vi "LEM_Paramters.vi"(8 "error in":errorcluster, 11 "Model Data":T2 {"Matricies"."K" format="%#_6e"; "Matricies"."Dout" format="%#_6e"; "Matricies"."Bout" format="%#_6e"; "Matricies"."Aout" format="%#_6e"; "Matricies"."Dint" format="%#_6e"; "Matricies"."Bint" format="%#_6e"; "Matricies"."Aint" format="%#_6e"; "Constants"."Z" format="%^#_6e"}) -> (0 "error out":errorcluster, 3 "Model Data Out":T2 {"Matricies"."K" format="%#_6e"; "Matricies"."Dout" format="%#_6e"; "Matricies"."Bout" format="%#_6e"; "Matricies"."Aout" format="%#_6e"; "Matricies"."Dint" format="%#_6e"; "Matricies"."Bint" format="%#_6e"; "Matricies"."Aint" format="%#_6e"; "Constants"."Z" format="%^#_6e"})   [LabVIEW 2022 SP3]
uses:
  Model Data.ctl
  PZT type.ctl
  Piezo_Discs.ctl
  LEM_Params.ctl
  Layer Properties.ctl
  Matricies.ctl
  <vilib>/Utility/error.llb/DialogType.ctl
  <vilib>/Analysis/2dsp.llb/Integral Method.ctl
  <vilib>/Analysis/8numeric.llb/1D Numeric Integration.vi
  <vilib>/Analysis/NI_AALPro.lvlib
panel:
  out "LEM Parameters":T1
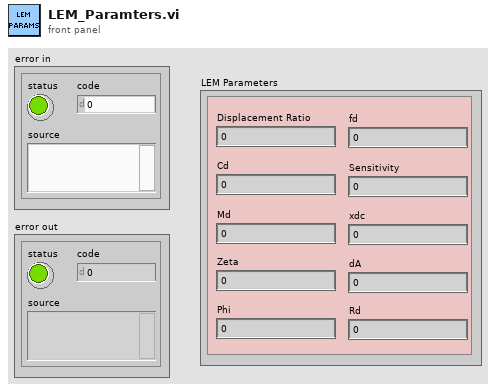
[diagram p1: front panel]
types:
  T1 = typedef "LEM_Params.ctl" = cluster{"Displacement Ratio":dbl, "Cd":dbl, "Md":dbl, "xdc":dbl, "fd":dbl, "Sensitivity":dbl, "dA":dbl, "Rd":dbl, "Zeta":dbl, "Phi":dbl}
  T2 = typedef "Model Data.ctl" = cluster{"Disc Properties":cluster{"Type":T3, "Disc Model":T4}, "Constants":cluster{"Radius":dbl[], "U(r)":dbl[], "W(r)":dbl[], "Vac":dbl, "P":dbl, "RiRo":dbl, "Area Density (r)":dbl[], "Ro":dbl, "Ri":dbl, "Z":dbl[], "Nr":dbl, "Mr":dbl, "c":dbl[], "AoC":dbl, "BoC":dbl, "AiC":dbl, "BiC":dbl, "f1":dbl, "f2":dbl}, "LEM Parameters":T1, "Layer Properties":T5[], "Matricies":T6}
  T3 = typedef "PZT type.ctl" = enum16{"Bimorph", "Unimorph"}
  T4 = typedef "Piezo_Discs.ctl" = enum16{"FTBD-21T-4.0A1", "PZT-5A (Gallas 1)", "PZT-5A (Gallas 2)", "AB4113B", "Create new disc...", "Load disc from file..."}
  T5 = typedef "Layer Properties.ctl" = cluster{"E":dbl, "R":dbl, "rho":dbl, "rhoA":dbl, "v":dbl, "A":dbl, "t":dbl, "d31":dbl, "size":enum16{"Outer", "Inner"}}
  T6 = typedef "Matricies.ctl" = cluster{"Aint":dbl[][], "Bint":dbl[][], "Dint":dbl[][], "Aout":dbl[][], "Bout":dbl[][], "Dout":dbl[][], "b":dbl[], "K":dbl[][]}
  T7 = typedef "DialogType.ctl" = u16
  T8 = typedef "NI_AALPro.lvlib/Integral Method.ctl" = i32
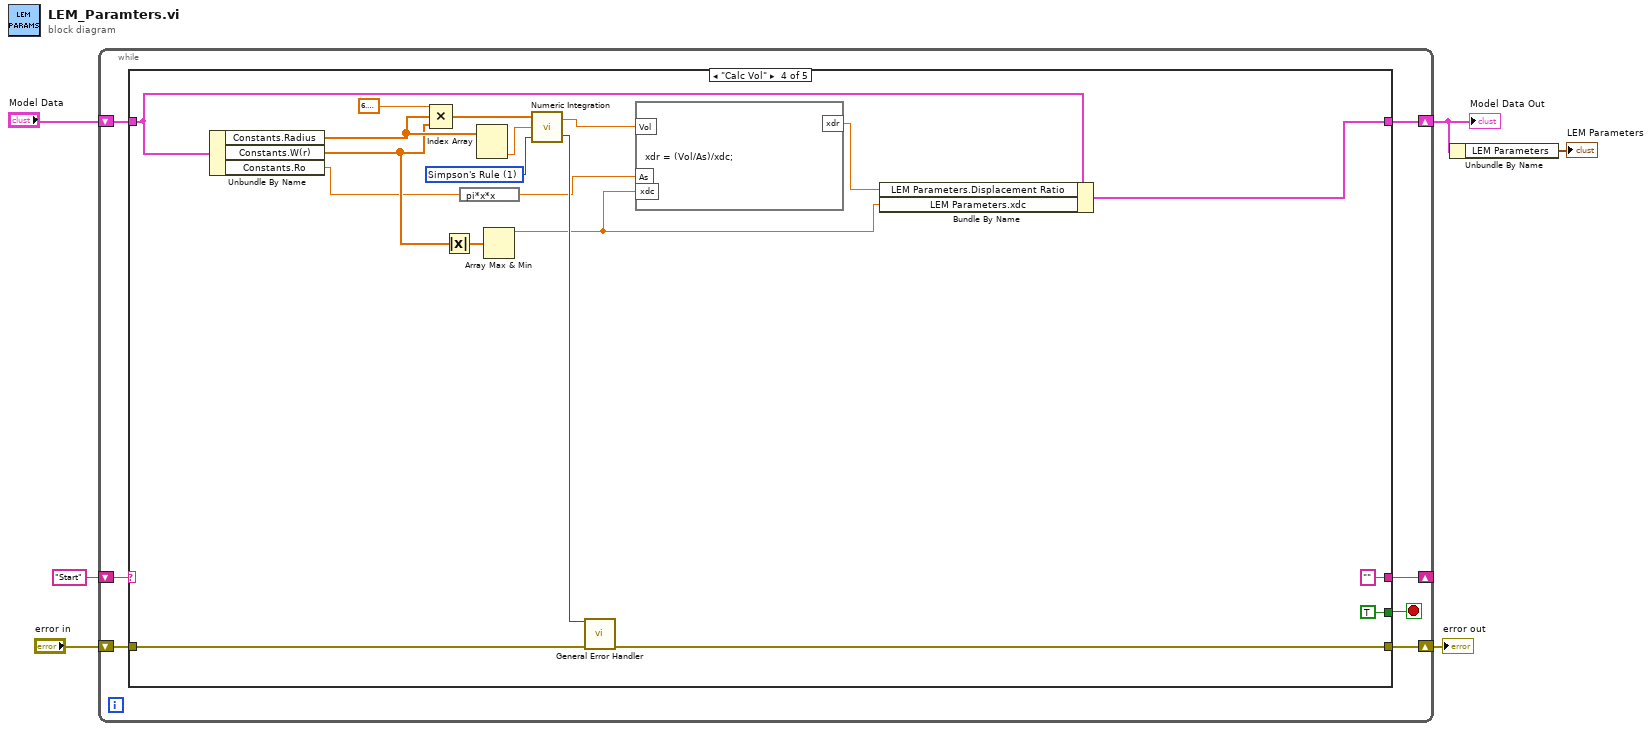
[diagram p0: block diagram]
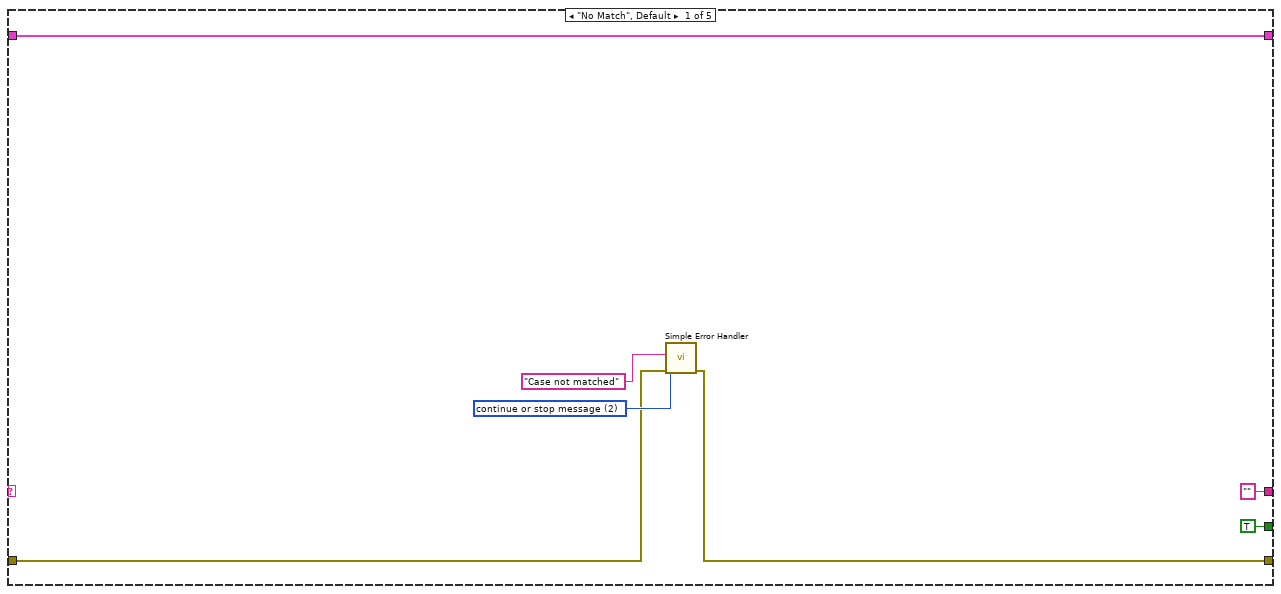
[diagram p2: hidden frame]
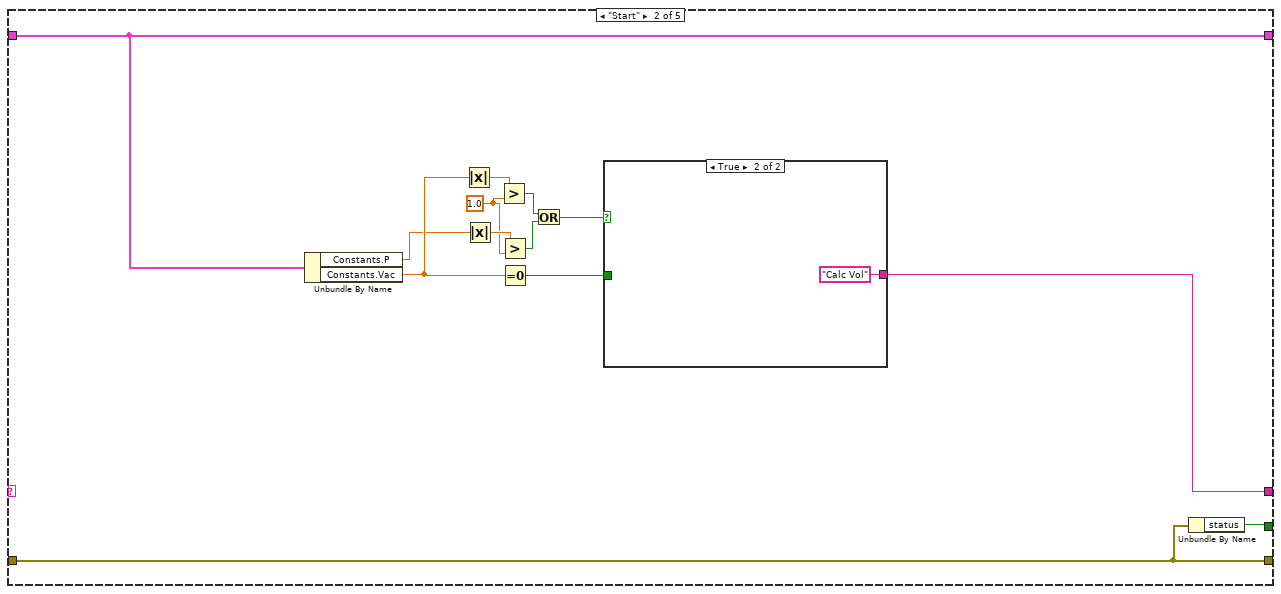
[diagram p3: hidden frame]
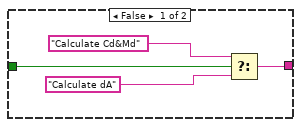
[diagram p4: hidden frame]
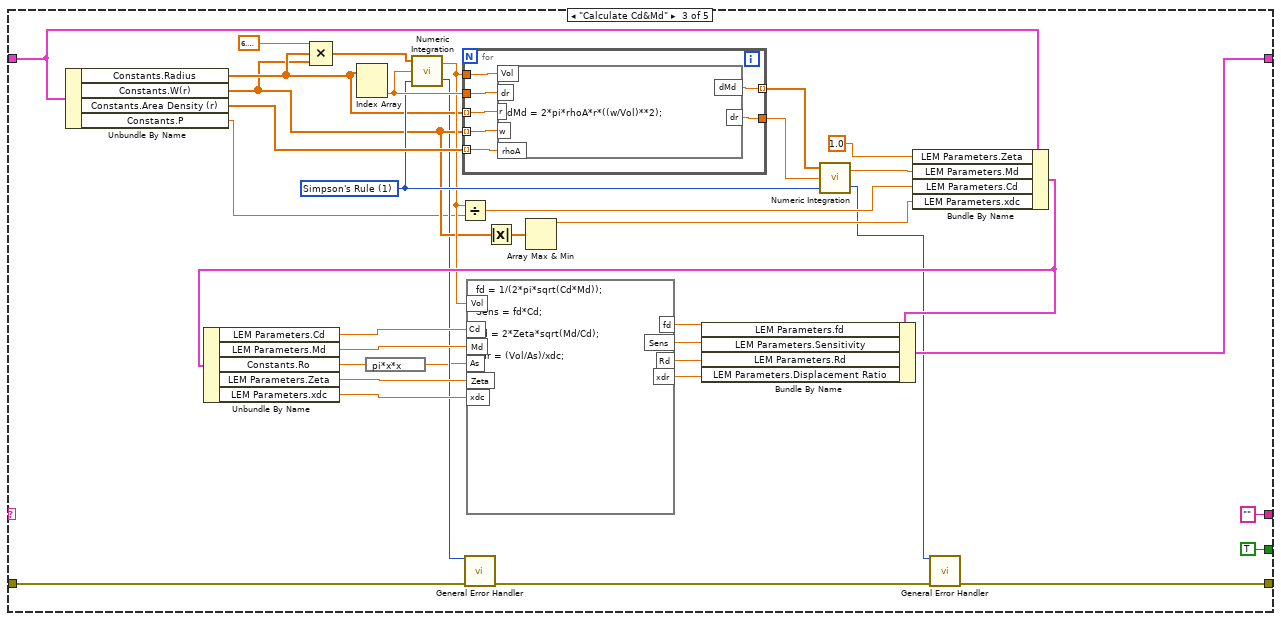
[diagram p5: hidden frame]
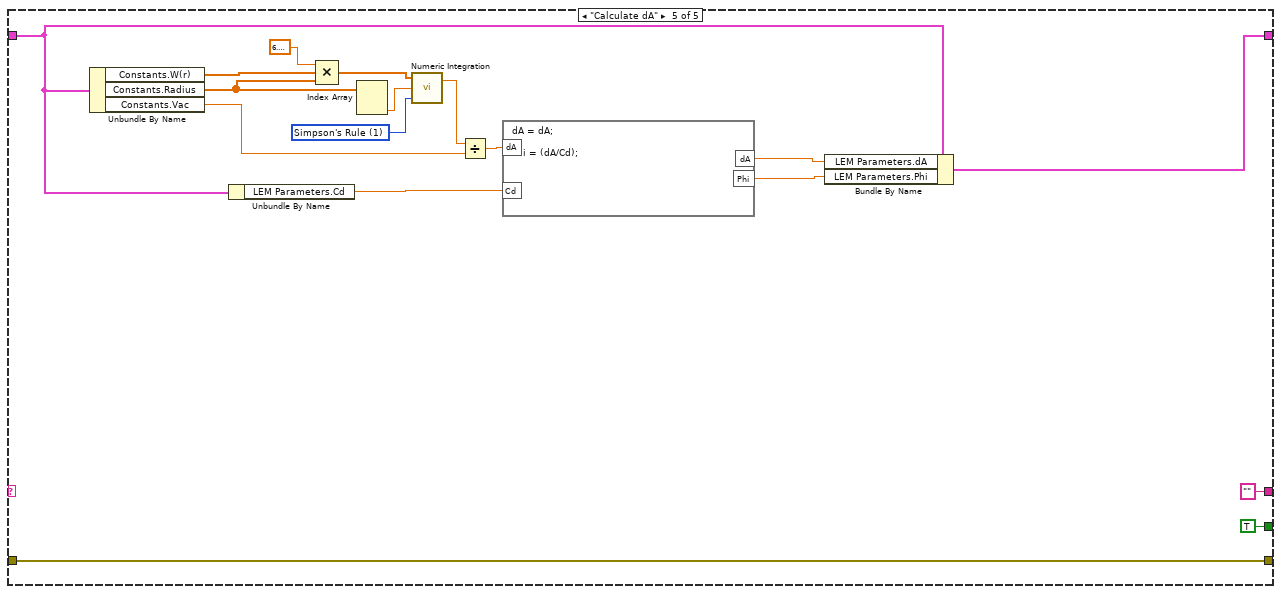
[diagram p6: hidden frame]
diagram:
  n1 = while {
    shift-right: [w12] -> w2
    shift-left: "Model Data" -> [w13]
    shift-right: [w9] -> _
    shift-left: "Start" -> [w11]
    shift-right: [w7] -> w4
    shift-left: "error in" -> [w8]
    stop <- w10 stop-if-true
    n2 = case shown="\"Calc Vol\"" w11 {
      tunnel: w13 -> [w18 w31 w74 w83 w109]
      tunnel: [w18 w31 w63 w96 w108] -> w12
      tunnel: [TRUE w29 TRUE TRUE TRUE] -> w10
      tunnel: ["" w32 "" "" ""] -> w9
      tunnel: w8 -> [w15 w30 w44 w89 w101]
      tunnel: [w14 w30 w42 w86 w101] -> w7
      frame "No Match", Default {
        w19 = T7 2 items=["no dialog", "OK message", "continue or stop message", "OK message + warnings", "continue/stop + warnings"] ("type of dialog (OK msg:1)")
        n3 = call <vilib>:"Simple Error Handler.vi"("error source (\" \")"="Case not matched", "type of dialog (OK msg:1)"=w19, "error in (no error)"=w15) -> ("error out"=w14:errorcluster)  [unwired: 2 in, 4 out]
      }
      frame "Start" {
        w24 = 1.0 ("y")
        n4 = Unbundle By Name(w31) -> ("Constants.P"=w25:dbl, "Constants.Vac"=w28:dbl)
        n5 = Absolute Value(x=w28) -> (abs(x)=w27:dbl)
        n6 = Absolute Value(x=w25) -> (abs(x)=w26:dbl)
        n7 = Greater?(x=w27, y=w24) -> (0:w23:bool)
        n8 = Greater?(x=w26, y=w24) -> (0:w22:bool)
        n9 = Equal To 0?(x=w28) -> (x = 0?=w33:bool)
        n10 = Or(x=w23, y=w22) -> (x .or. y?=w21:bool)
        n11 = case shown="True" w21 {
          tunnel: w33 -> [w37 _]
          tunnel: [w36 "Calc Vol"] -> w32
          frame False {
            n12 = Select(t="Calculate Cd&Md", s=w37, f="Calculate dA") -> (s? t:f=w36:string)
          }
          frame True {
          }
        }
        n13 = Unbundle By Name(w30) -> ("status"=w29:bool)
      }
      frame "Calculate Cd&Md" {
        w65 = T8 1 items=["Trapezoidal Rule", "Simpson's Rule", "Simpson's 3/8 Rule", "Bode Rule"] ("integration method")
        n14 = Unbundle By Name(w74) -> ("Constants.Radius"=w52:dbl[], "Constants.W(r)"=w48:dbl[], "Constants.Area Density (r)"=w70:dbl[], "Constants.P"=w40:dbl)
        n15 = Compound Arithmetic op=MULTIPLY(6.283185307179586, w52, w48) -> (w50:dbl[])
        n16 = Index Array(array=w52) -> (element #2=w71:dbl)  [unwired: 2 in, 1 out]
        n17 = call-poly <vilib>:"Numeric Integration.vi"("integration method"=w65, "dt"=w71, "Input Array"=w50) -> ("error"=w45:i32, "result"=w55:dbl)
        n18 = Divide(x=w55, y=w40) -> (x/y=w67:dbl)
        n19 = for {
          tunnel: w52 -> [w81] mode=indexing
          tunnel: w48 -> [w80] mode=indexing
          tunnel: w55 -> [w79]
          tunnel: [w78] -> w69 mode=indexing
          tunnel: w71 -> [w77]
          tunnel: [w76] -> w68
          tunnel: w70 -> [w75] mode=indexing
          n20 = formula code="dMd = 2*pi*rhoA*r*((w/Vol)**2);"("r"=w81, "w"=w80, "Vol"=w79, "rhoA"=w75, "dr"=w77) -> ("dMd"=w78:dbl, "dr"=w76:dbl)
        }
        n21 = call <vilib>:"General Error Handler.vi"("[error code] (0)"=w45, "error in (no error)"=w44) -> ("error out"=w43:errorcluster)  [unwired: 9 in, 4 out]
        n22 = Absolute Value(x=w48) -> (abs(x)=w39:dbl[])
        n23 = Array Max & Min(array=w39) -> (max value=w47:dbl)  [unwired: 3 out]
        n24 = call-poly <vilib>:"Numeric Integration.vi"("integration method"=w65, "dt"=w68, "Input Array"=w69) -> ("error"=w46:i32, "result"=w66:dbl)
        n25 = Bundle By Name(cluster=w74, "LEM Parameters.Zeta"=1.0, "LEM Parameters.Md"=w66, "LEM Parameters.Cd"=w67, "LEM Parameters.xdc"=w47) -> (w64:T2)
        n26 = Unbundle By Name(w64) -> ("LEM Parameters.Cd"=w62:dbl, "LEM Parameters.Md"=w61:dbl, "Constants.Ro"=w60:dbl, "LEM Parameters.Zeta"=w53:dbl, "LEM Parameters.xdc"=w49:dbl)
        n27 = expression code="pi*x*x"(w60) -> (w41:dbl)
        n28 = formula code="fd = 1/(2*pi*sqrt(Cd*Md));\n\nSens = fd*Cd;\n\nRd = 2*Zeta*sqrt(Md/Cd);\n\nxdr = (Vol/As)/xdc;"("As"=w41, "Cd"=w62, "Md"=w61, "Vol"=w55, "Zeta"=w53, "xdc"=w49) -> ("fd"=w59:dbl, "Sens"=w58:dbl, "Rd"=w56:dbl, "xdr"=w54:dbl)
        n29 = Bundle By Name(cluster=w64, "LEM Parameters.fd"=w59, "LEM Parameters.Sensitivity"=w58, "LEM Parameters.Rd"=w56, "LEM Parameters.Displacement Ratio"=w54) -> (w63:T2)
        n30 = call <vilib>:"General Error Handler.vi"("[error code] (0)"=w46, "error in (no error)"=w43) -> ("error out"=w42:errorcluster)  [unwired: 9 in, 4 out]
      }
      frame "Calc Vol" {
        w97 = T8 1 items=["Trapezoidal Rule", "Simpson's Rule", "Simpson's 3/8 Rule", "Bode Rule"] ("integration method")
        n31 = Unbundle By Name(w83) -> ("Constants.Radius"=w94:dbl[], "Constants.W(r)"=w91:dbl[], "Constants.Ro"=w85:dbl)
        n32 = Compound Arithmetic op=MULTIPLY(6.283185307179586, w94, w91) -> (w92:dbl[])
        n33 = Absolute Value(x=w91) -> (abs(x)=w87:dbl[])
        n34 = expression code="pi*x*x"(w85) -> (w88:dbl)
        n35 = Index Array(array=w94) -> (element #2=w98:dbl)  [unwired: 2 in, 1 out]
        n36 = Array Max & Min(array=w87) -> (max value=w84:dbl)  [unwired: 3 out]
        n37 = call-poly <vilib>:"Numeric Integration.vi"("integration method"=w97, "dt"=w98, "Input Array"=w92) -> ("error"=w90:i32, "result"=w95:dbl)
        n38 = call <vilib>:"General Error Handler.vi"("[error code] (0)"=w90, "error in (no error)"=w89) -> ("error out"=w86:errorcluster)  [unwired: 9 in, 4 out]
        n39 = formula code="xdr = (Vol/As)/xdc;"("As"=w88, "Vol"=w95, "xdc"=w84) -> ("xdr"=w82:dbl)
        n40 = Bundle By Name(cluster=w83, "LEM Parameters.Displacement Ratio"=w82, "LEM Parameters.xdc"=w84) -> (w96:T2)
      }
      frame "Calculate dA" {
        w113 = T8 1 items=["Trapezoidal Rule", "Simpson's Rule", "Simpson's 3/8 Rule", "Bode Rule"] ("integration method")
        n41 = Unbundle By Name(w109) -> ("Constants.W(r)"=w104:dbl[], "Constants.Radius"=w103:dbl[], "Constants.Vac"=w114:dbl)
        n42 = Unbundle By Name(w109) -> ("LEM Parameters.Cd"=w111:dbl)
        n43 = Compound Arithmetic op=MULTIPLY(6.283185307179586, w104, w103) -> (w102:dbl[])
        n44 = Index Array(array=w103) -> (element #2=w115:dbl)  [unwired: 2 in, 1 out]
        n45 = call-poly <vilib>:"Numeric Integration.vi"("integration method"=w113, "dt"=w115, "Input Array"=w102) -> ("result"=w112:dbl)  [unwired: 1 out]
        n46 = Divide(x=w112, y=w114) -> (x/y=w110:dbl)
        n47 = formula code="dA = dA;\n\nPhi = (dA/Cd);"("Cd"=w111, "dA"=w110) -> ("dA"=w107:dbl, "Phi"=w106:dbl)
        n48 = Bundle By Name(cluster=w109, "LEM Parameters.dA"=w107, "LEM Parameters.Phi"=w106) -> (w108:T2)
      }
    }
  }
  "error out" <- w4
  "Model Data Out" <- w2
  n49 = Unbundle By Name(w2) -> ("LEM Parameters"=→"LEM Parameters":T1)
